vi "Read Device Information.vi"(8 "error in (no error)":errorcluster, 11 "TwinCAT ADS in":refnum<class "TwinCAT ADS.lvclass">) -> (0 "error out":errorcluster, 1 "Device Information":T1, 3 "TwinCAT ADS out":refnum<class "TwinCAT ADS.lvclass">)   [LabVIEW 2018, in "TwinCAT ADS.lvclass"]
uses:
  TwinCAT ADS.lvclass
  Controls/Device Information.ctl
  TwinCAT ADS.lvclass/TwinCAT ADS.ctl
  TwinCAT.Ads
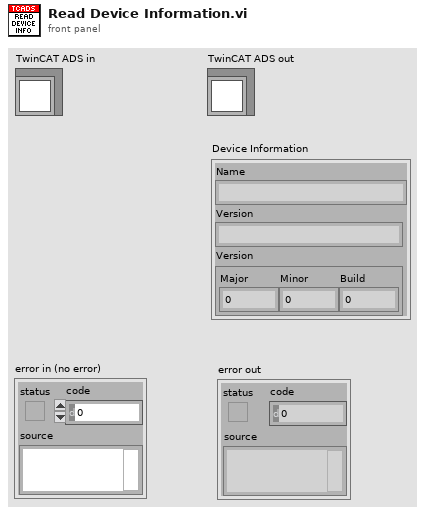
[diagram p1: front panel]
types:
  T1 = typedef "TwinCAT ADS.lvclass/Device Information.ctl" = cluster{"Name":string, "Version":string, "Version":cluster{"Major":i32, "Minor":i32, "Build":i32}}
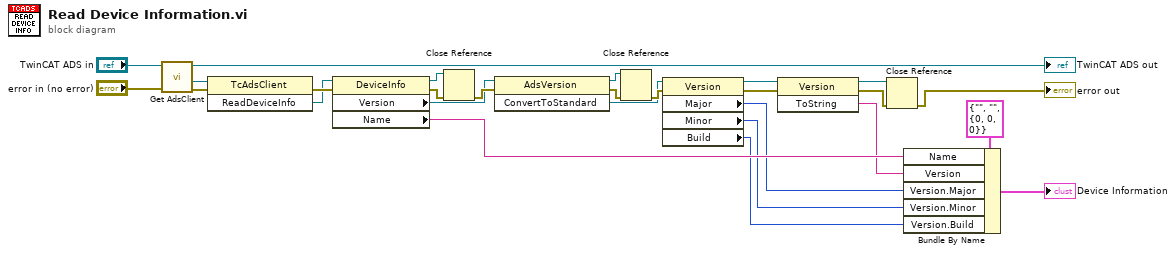
[diagram p0: block diagram]
diagram:
  n1 = call "Get AdsClient.vi"("error in (no error)"="error in (no error)", "TwinCAT ADS in"="TwinCAT ADS in") -> ("error out"=w11:errorcluster, ".NET TcAdsClient"=w7:refnum<k24>, "TwinCAT ADS out"=→"TwinCAT ADS out":refnum<class "TwinCAT ADS.lvclass">)  [unwired: 7 in]
  n2 = invoke class="TcAdsClient" method="ReadDeviceInfo"(reference=w7, error in=w11) -> (error out=w22:errorcluster, "ReadDeviceInfo"=w21:refnum<k24>)  [unwired: 1 in, 1 out]
  n3 = property class="DeviceInfo"(reference=w21, error in=w22) -> (reference out=w8:refnum<k24>, error out=w9:errorcluster, "Version"=w20:refnum<k24>, "Name"=w15:string)
  n4 = Close Reference(reference=w8, error in (no error)=w9) -> (error out=w26:errorcluster)
  n5 = invoke class="AdsVersion" method="ConvertToStandard"(reference=w20, error in=w26) -> (reference out=w5:refnum<k24>, error out=w6:errorcluster, "ConvertToStandard"=w19:refnum<k24>)  [unwired: 1 in]
  n6 = Close Reference(reference=w5, error in (no error)=w6) -> (error out=w27:errorcluster)
  n7 = property class="Version"(reference=w19, error in=w27) -> (reference out=w17:refnum<k24>, error out=w18:errorcluster, "Major"=w13:i32, "Minor"=w12:i32, "Build"=w1:i32)
  n8 = invoke class="Version" method="ToString"(reference=w17, error in=w18) -> (reference out=w3:refnum<k24>, error out=w4:errorcluster, "ToString"=w14:string)  [unwired: 1 in]
  n9 = Close Reference(reference=w3, error in (no error)=w4) -> (error out=→"error out":errorcluster)
  n10 = Bundle By Name(cluster=T1 {"Name"="", "Version"="", "Version"={"Major"=0, "Minor"=0, "Build"=0}} ("Device Infomation"), "Name"=w15, "Version"=w14, "Version.Major"=w13, "Version.Minor"=w12, "Version.Build"=w1) -> (→"Device Information":T1)
